vi "_PC_Daemon_MathieuEqCalc.vi"(8 "error in (no error)":errorcluster) -> (0 "error out":errorcluster)   [LabVIEW 2018]
uses:
  PublicSubVI/Ctl/MathieuEqParam.ctl
  <vilib>/event_ctls.llb/eventvkey.ctl
panel:
  in  "Target":enum16{"m/z", "Volt", "Freq", "Beta"}(ring)=enum."Freq"
  in  "Calc":bool
  in  "Parametres":T1={"mz(Th)"=0.0, "Amp(V)"=330.0, "Freq(Hz)"=0.0, "Beta"=1.0, "r_0 (mm)"=10.0, "z_0 (mm)"=7.07} {"z_0 (mm)" format="%#.3f"; "r_0 (mm)" format="%#.3f"; "Beta" format="%#_5f"; "Freq(Hz)" format="%#.2f"; "Amp(V)" format="%#.2f"; "mz(Th)" format="%#_6f"}
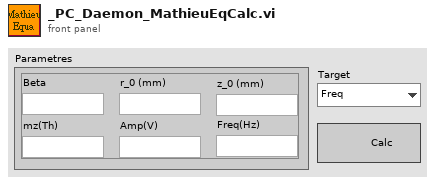
[diagram p1: front panel]
types:
  T1 = typedef "MathieuEqParam.ctl" = cluster{"mz(Th)":ext, "Amp(V)":ext, "Freq(Hz)":ext, "Beta":ext, "r_0 (mm)":ext, "z_0 (mm)":ext}
  T2 = typedef "eventvkey.ctl" = enum16{"ASCII", "Enter", "Return", "Shift", "Ctrl", "Alt", "Cmd", "Opt", "Caps", "NumLock", "Clear", "Break", "Up", "Down", "Left", "Right", "Insert", "Delete", "Home", "End", "PageUp", "PageDown", "Escape", "Help", "Pause", "ScrollLock", "F1", "F2", "F3", "F4", "F5", "F6", "F7", "F8", "F9", "F10", "F11", "F12", "F13", "F14", "F15", "F16", "F17", "F18", "F19", "F20", "F21", "F22", "F23", "F24", "Play", "VolumeUp", "VolumeDown", "Mute", "Two Byte Char"}
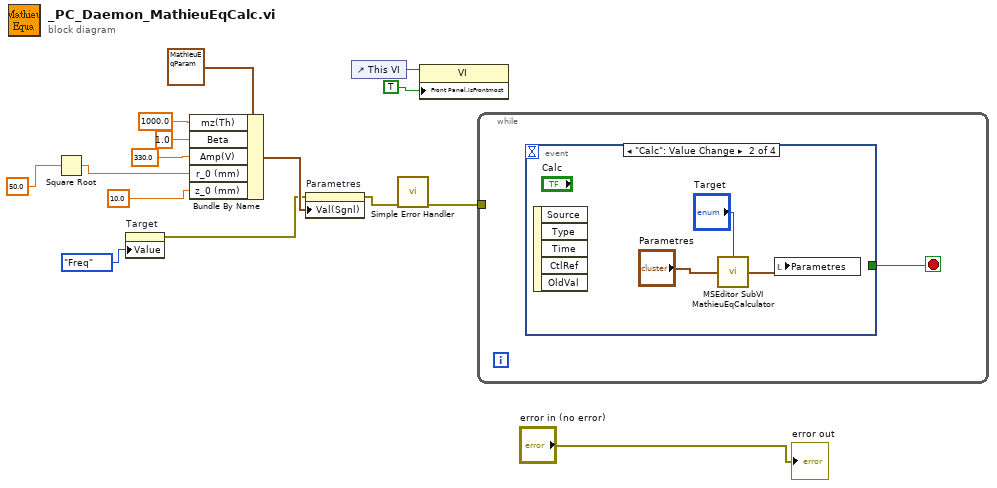
[diagram p0: block diagram]
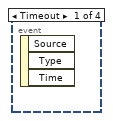
[diagram p2: hidden frame]
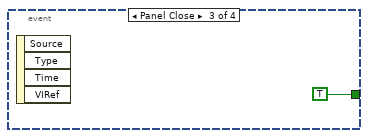
[diagram p3: hidden frame]
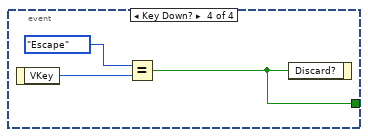
[diagram p4: hidden frame]
diagram:
  n1 = Square Root(x=50.0) -> (sqrt(x)=w2:dbl)
  n2 = property on="Target" class="Enum (strict)"("Value"=enum16{"m/z", "Volt", "Freq", "Beta"}."Freq" ("Target")) -> (error out=w8:errorcluster)  [unwired: 2 in, 1 out]
  n3 = Bundle By Name(cluster=T1 {"mz(Th)"=0.0, "Amp(V)"=330.0, "Freq(Hz)"=0.0, "Beta"=0.908046, "r_0 (mm)"=10.0, "z_0 (mm)"=7.07} ("Value (Signaling)"), "mz(Th)"=1000.0, "Beta"=1.0, "Amp(V)"=330.0, "r_0 (mm)"=w2, "z_0 (mm)"=10.0) -> (w13:T1)
  n4 = property on="Parametres" class="Clust (strict)"(error in=w8, "Val(Sgnl)"=w13) -> (error out=w12:errorcluster)  [unwired: 1 in, 1 out]
  n5 = control-ref of="This VI"() -> (w10:refnum<vi>)
  n6 = call <vilib>:"Simple Error Handler.vi"("error in (no error)"=w12) -> ("error out"=w11:errorcluster)  [unwired: 4 in, 4 out]
  n7 = property class="VI"(reference=w10, "Front Panel.IsFrontmost"=TRUE) -> ()  [unwired: 1 in, 2 out]
  n8 = while {
    tunnel: w11 -> [_]
    stop <- w16 stop-if-true
    n9 = event shown="[1] \"Calc\": Value Change" {
      selector: _ -> [_ _ _ _]
      dyn-events: _ -> [_ _ _ _]
      timeout: _ -> [_ _ _ _]
      tunnel: [_ _ TRUE w21] -> w16
      event Timeout {
        n10 = event-data() -> ()  [unwired: 1 in, 3 out]
      }
      event "Calc": Value Change {
        n11 = event-data() -> ()  [unwired: 1 in, 5 out]
        n12 = call "MSEditor SubVI MathieuEqCalculator.vi"("Target (Freq)"="Target", "Parametres in"="Parametres") -> ("Parametres out"=w18:T1)  [unwired: 2 in]
        n13 = local write "Parametres"(w18) -> ()
      }
      event Panel Close {
        n14 = event-data() -> ()  [unwired: 1 in, 4 out]
      }
      event Key Down? {
        n15 = event-data() -> ("VKey"=w23:T2)  [unwired: 1 in]
        n16 = Equal?(x=eventvkey."Escape", y=w23) -> (x = y?=w21:bool)
        n17 = event-data("Discard?"=w21) -> ()  [unwired: 1 in, 1 out]
      }
    }
  }
  "error out" <- "error in (no error)"
